vi "Process_BRAM_data.vi"(0 "Frame_data":u8[](array[numeric])) -> (10 "BRAM_hist_out":u16[][](array[numeric]))   [LabVIEW 2019]
panel:
  out "sum":u16
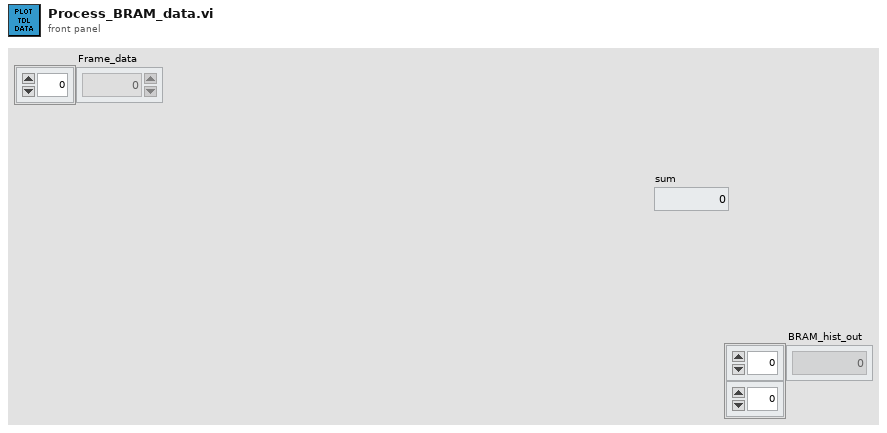
[diagram p1: front panel]
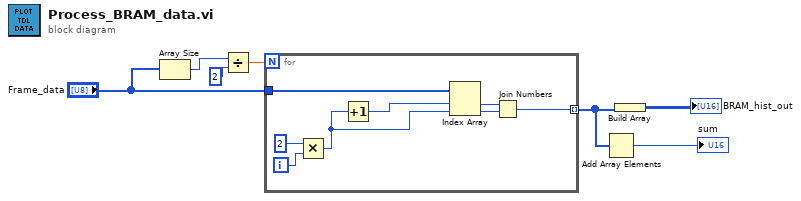
[diagram p0: block diagram]
diagram:
  n1 = Array Size(array="Frame_data") -> (size(s)=w4:i32)
  n2 = Divide(x=w4, y=2) -> (x/y=w5:dbl)
  n3 = for {
    N: w5 -> [_]
    tunnel: "Frame_data" -> [w15]
    tunnel: [w10] -> w2 mode=indexing
    i -> [w14]
    n4 = Multiply(x=2, y=w14) -> (x*y=w12:i32)
    n5 = Increment(x=w12) -> (x+1=w11:i32)
    n6 = Index Array(array=w15, index #1=w11, index #2=w12) -> (element #1=w8:u8, element #2=w9:u8)
    n7 = Join Numbers(hi=w8, lo=w9) -> ((hi.lo)=w10:u16)
  }
  n8 = Add Array Elements(numeric array=w2) -> (sum=→"sum":u16)
  n9 = Build Array(w2) -> (→"BRAM_hist_out":u16[][])
